vi "Collect.vi"(8 "error in (no error)":errorcluster, 11 "Metric in":refnum<class "Metric.lvclass">) -> (0 "error out":errorcluster, 2 "Metrics":refnum<data-value>[](array[refnum]), 3 "Metric out":refnum<class "Metric.lvclass">)   [LabVIEW 2020, in "Metrics.lvlib" / "Metric.lvclass"]
uses:
  Metric.lvclass
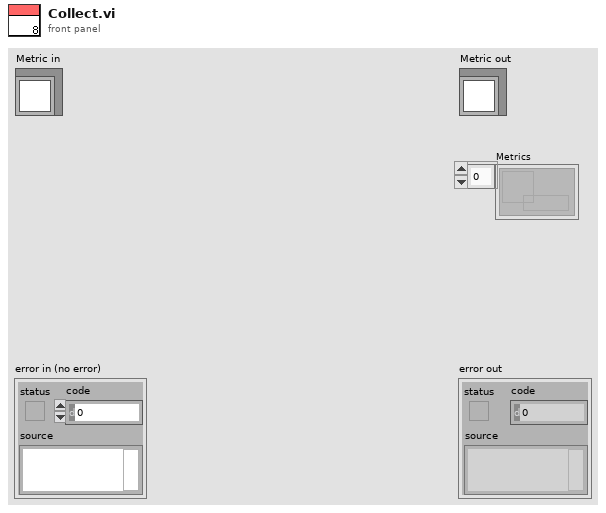
[diagram p1: front panel]
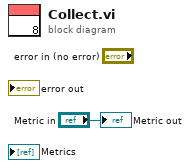
[diagram p0: block diagram]
diagram:
  "Metric out" <- "Metric in"
